vi "RT Loop - Log video.vi"(8 "error in (no error)":errorcluster, 9 "Acceleration RT FIFO In":T1, 11 "Message Queue":refnum<queue>) -> ()   [LabVIEW 2017]
doc: "Receive triggered data from Analyze Acceleration Loop and log the data to disk."
uses:
  support/Message Queue/Message Cluster.ctl
  controls/Acceleration RT FIFO Reference.ctl
  Globals/Global - All RT Loop Stop.vi
  Globals/Global - Configuration Options.vi
  support/Logging/Logging.lvlib
  support/Message Queue/Message Queue.lvlib
panel:
  out "Acceleration Log Folder":path=path "/home/lvuser/Log/logfiles_deploy"
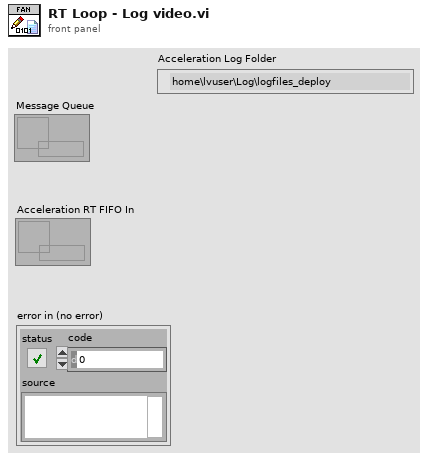
[diagram p1: front panel]
types:
  T1 = typedef "Acceleration RT FIFO Reference.ctl" = refnum<k33>
  T2 = typedef "IMAQ Image.ctl" = refnum<image>
  T3 = typedef "IMAQ AVI2 Refnum.ctl" = refnum<k20>
  T4 = typedef "IMAQdx.ctl" = refnum<k21>
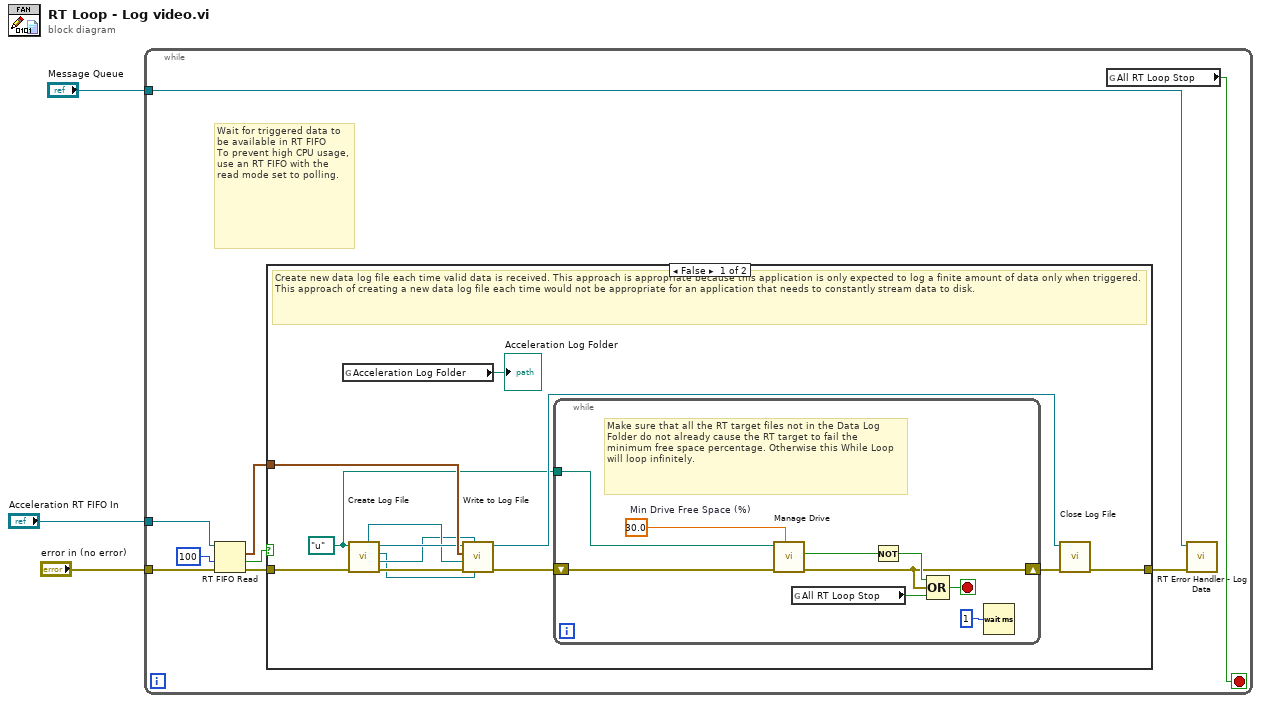
[diagram p0: block diagram]
diagram:
  n1 = while {
    tunnel: "Acceleration RT FIFO In" -> [w10]
    tunnel: "Message Queue" -> [w6]
    tunnel: "error in (no error)" -> [w12]
    stop <- w7 stop-if-true
    # "Wait for triggered data to be available in RT FIFO\nTo prevent high CPU usage, use an RT FIFO with the read mode set to polling."
    n2 = RT FIFO Read(0:w10, 2:100 ("ms timeout (0)"), 3:w12) -> (9:w8:waveform(dbl)[], 10:w4:bool, 11:w11:errorcluster)  [unwired: 1 in, 2 out]
    n3 = case shown="False" w4 {
      tunnel: w8 -> [w25 _]
      tunnel: w11 -> [w20 w35]
      tunnel: [w22 w35] -> w5
      frame False {
        w17 = path "u:/" ("file path (use dialog)")
        # "Create new data log file each time valid data is received. This approach is appropriate because this application is only expected to log a finite amount of data only when triggered.  This approach of creating a new data log file each time would not be appropriate for an application that needs to constantly stream data to disk."
        n4 = global read "Global - Configuration Options.vi" "Acceleration Log Folder"() -> (→"Acceleration Log Folder":path)
        n5 = call "Create Log File.vi"("error in (no error)"=w20, "Acceleration Exceeded Log Folder"=w17) -> ("error out"=w21:errorcluster, "New Image"=w14:T2, "AVI Refnum"=w13:T3, "Log File out"=w19:refnum<k34>, "Session Out"=w15:T4)  [unwired: 5 in]
        n6 = call "Write to Log File.vi"("AVI Refnum"=w13, "New Image"=w14, "error in (no error)"=w21, "Session Out"=w15, "Array of Waveforms"=w25, "Log File in"=w19) -> ("error out"=w24:errorcluster, "Log File out"=w18:refnum<k34>)  [unwired: 4 in]
        n7 = while {
          shift-right: [w29] -> w23
          shift-left: w24 -> [w30]
          tunnel: w17 -> [w27]
          stop <- w34 stop-if-true
          w28 = 30.0  # Min Drive Free Space (%)
          # "Make sure that all the RT target files not in the Data Log Folder do not already cause the RT target to fail the minimum free space percentage. Otherwise this While Loop will loop infinitely."
          n8 = call "Manage Drive.vi"("Min Drive Free Space (%)"=w28, "error in"=w30, "Data Folder"=w27) -> ("error out"=w29:errorcluster, "Drive Space Below Limit"=w26:bool)  [unwired: 7 in]
          n9 = global read "Global - All RT Loop Stop.vi" "All RT Loop Stop"() -> (w31:bool)
          n10 = Not(x=w26) -> (.not. x?=w33:bool)
          n11 = Compound Arithmetic op=OR(w33, w29, w31) -> (w34:bool)
          n12 = Wait (ms)(milliseconds to wait=u32 1) -> ()  [unwired: 1 out]
        }
        n13 = call "Close Log File.vi"("error in (no error)"=w23, "tdms file"=w18) -> ("error out"=w22:errorcluster)  [unwired: 9 in]
      }
      frame True {
        # "Timed out - No data"
      }
    }
    n14 = global read "Global - All RT Loop Stop.vi" "All RT Loop Stop"() -> (w7:bool)
    n15 = call "RT Error Handler - Log Data.vi"("error in (no error)"=w5, "Message Queue"=w6) -> ()  [unwired: 9 in, 1 out]
  }
